vi "BS the tug main A.vi"() -> ()   [LabVIEW 2012]
uses:
  <vilib>/userdefined/High Color/IMAQdx.ctl
  <vilib>/vision/driver/NI_Vision_Acquisition_Software.lvlib
  <vilib>/vision/NI_Vision_Development_Module.lvlib
panel:
  out "Scaled image":T1(plugin-control)
  out "Running?":bool
  out "All found?":bool
  in  "Data sent":string
  out "error out":errorcluster
  out "Image":T1(plugin-control)
  in  "stop":bool
  in  "Image Type":T2 items=["Grayscale (U8)", "Grayscale (I16)", "Grayscale (SGL)", "Complex (CSG)", "RGB (U32)", "HSL (U32)", "RGB (U64)", "Grayscale (U16)"]
  in  "Session In":T3="cam0"
  # "This VI receives an image from the camera above the pool and modifies the image to be 1032 x 1032 it then:\n1. Locates (4) tugs with greek letter symbols\n2. Locates (4) buoys with circle symbols\n3. Records the time the image is taken\n4. Creates a single string of that data and transmits the string using UDP to port 61557\n\nTO OPERATE START THE ROUTINE!"
  # "The Point Grey camera settings should be:\nAuto Exposure      Auto\nBrightness             Relative     200\nGain                       Auto\nFrame Rate           Absolute   20\nShutter                  Auto\n\nThese values are programmed into this VI\n\nThe overhead lights should be OFF"
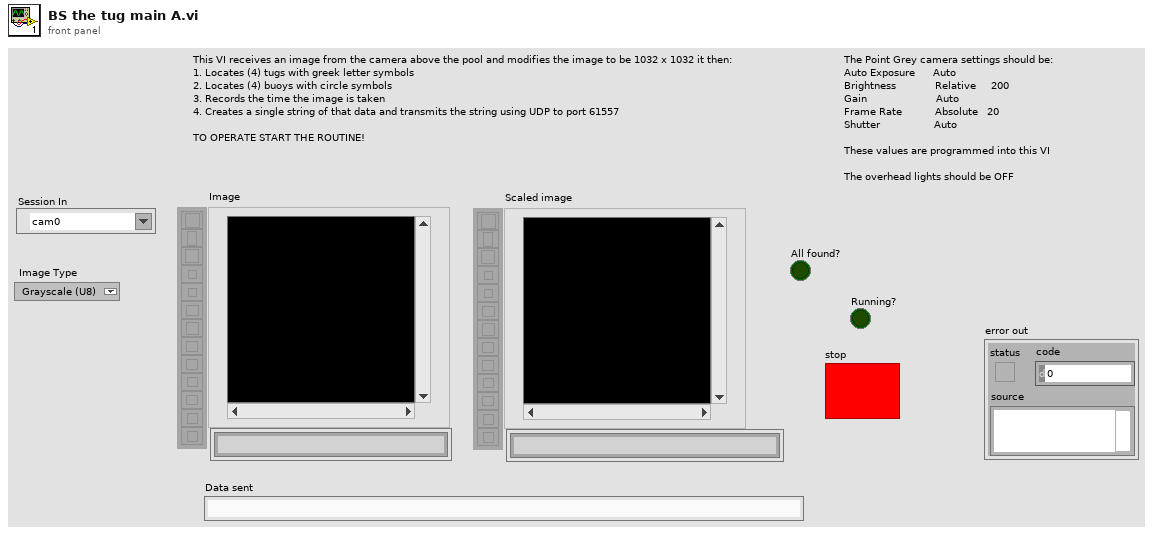
[diagram p1: front panel]
types:
  T1 = typedef "IMAQ Image.ctl" = refnum<image>
  T2 = typedef "Image Type" = u32
  T3 = typedef "IMAQdx.ctl" = refnum<k21>
  T4 = cluster{"Greek Letter":string, i16, i16, i16, bool}[]
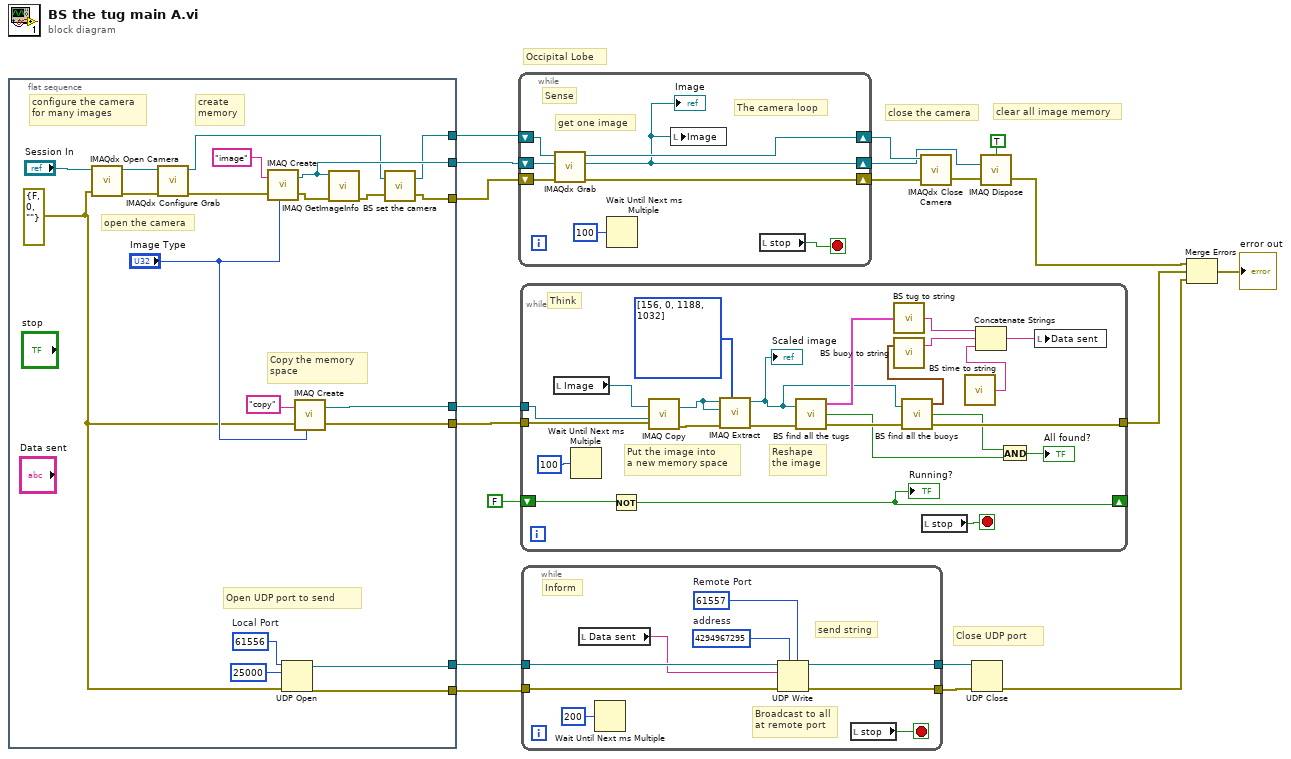
[diagram p0: block diagram]
diagram:
  # "Occipital Lobe"
  # "Close UDP port"
  # "clear all image memory"
  # "close the camera"
  n1 = flat-sequence {
    tunnel: [w22] -> w12
    tunnel: [w20] -> w13
    tunnel: [w33] -> w14
    tunnel: [w30] -> w10
    tunnel: [w29] -> w11
    tunnel: [w26] -> w4
    tunnel: [w25] -> w3
    frame #0 {
      w28 = u16 61556  # Local Port
      w24 = errorcluster {"status"=FALSE, "code"=0, "source"=""} ("error in")
      # "Open UDP port to send"
      # "Copy the memory\nspace"
      # "create\nmemory"
      # "configure the camera\nfor many images"
      # "open the camera"
      n2 = call <vilib>:"IMAQdx Open Camera.vi"("error in"=w24, "Session In"="Session In") -> ("error out"=w36:errorcluster, "Session Out"=w37:T3)  [unwired: 1 in, 7 out]
      n3 = call <vilib>:"IMAQdx Configure Grab.vi"("error in"=w36, "Session In"=w37) -> ("error out"=w38:errorcluster, "Session Out"=w21:T3)  [unwired: 8 out]
      n4 = call "IMAQ Create"("Image Name"="image", "Image Type"="Image Type", "error in (no error)"=w38) -> ("New Image"=w33:T1, "error out"=w39:errorcluster)  [unwired: 1 in, 1 out]
      n5 = UDP Open(8:w24, 9:25000 ("timeout ms (25000)"), 11:w28) -> (port=w25:refnum<k16>, 0:w26:errorcluster)  [unwired: 3 out]
      n6 = call "IMAQ Create"("Image Name"="copy", "Image Type"="Image Type", "error in (no error)"=w24) -> ("New Image"=w29:T1, "error out"=w30:errorcluster)  [unwired: 2 in]
      n7 = call "IMAQ GetImageInfo"("error in (no error)"=w39, "Image"=w33) -> ("error out"=w23:errorcluster)  [unwired: 2 in, 7 out]
      n8 = call "BS set the camera.vi"("error in"=w23, "IMAQdx Session input"=w21) -> ("error out"=w22:errorcluster, "IMAQdx Session output"=w20:T3)
    }
  }
  n9 = while {
    shift-right: [w44] -> w19
    shift-left: w13 -> [w47]
    shift-right: [w40] -> w16
    shift-left: w14 -> [w46]
    shift-right: [w43] -> w18
    shift-left: w12 -> [w45]
    stop <- w41 stop-if-true
    # "Sense"
    # "The camera loop"
    # "get one image"
    n10 = call <vilib>:"IMAQdx Grab.vi"("error in"=w45, "Image In"=w46, "Session In"=w47) -> ("error out"=w43:errorcluster, "Image Out"=w40:T1, "Session Out"=w44:T3)  [unwired: 5 in, 1 out]
    "Image" <- w40
    n11 = Wait Until Next ms Multiple(millisecond multiple=u32 100) -> ()  [unwired: 1 out]
    n12 = local write "Image"(w40) -> ()
    n13 = local read "stop"() -> (w41:bool)
  }
  n14 = while {
    tunnel: w11 -> [w66]
    tunnel: w10 -> [w67]
    tunnel: [w56] -> w8
    shift-right: [w59] -> _
    shift-left: FALSE -> [w60]
    stop <- w62 stop-if-true
    # "Think"
    # "Reshape\nthe image"
    # "Put the image into \na new memory space"
    n15 = local read "Image"() -> (w65:T1)
    n16 = Wait Until Next ms Multiple(millisecond multiple=u32 100) -> ()  [unwired: 1 out]
    n17 = Not(x=w60) -> (.not. x?=w59:bool)
    "Running?" <- w59
    n18 = call "IMAQ Copy"("error in (no error)"=w67, "Image Dst"=w66, "Image Src"=w65) -> ("error out"=w69:errorcluster, "Image Dst Out"=w70:T1)  [unwired: 3 in]
    n19 = call "IMAQ Extract"("Optional Rectangle"=i32[] [156, 0, 1188, 1032], "error in (no error)"=w69, "Image Dst"=w70, "Image Src"=w70) -> ("error out"=w64:errorcluster, "Image Dst Out"=w57:T1)  [unwired: 6 in]
    "Scaled image" <- w57
    n20 = call "BS find all the tugs.vi"("Image Src"=w57, "error in"=w64) -> ("Tug location array"=w63:T4, "All found?"=w52:bool, "error out"=w58:errorcluster)
    n21 = call "BS tug to string.vi"("Tug location array"=w63) -> ("tug location string"=w51:string)
    n22 = call "BS find all the buoys.vi"("Image Src"=w57, "error in"=w58) -> ("Buoy Array"=w54:cluster{i16, i16}[], "Buoys found?"=w53:bool, "error out"=w56:errorcluster)
    n23 = call "BS buoy to string.vi"("Buoy Array"=w54) -> ("Buoy location string"=w50:string)  [unwired: 1 in, 1 out]
    n24 = local read "stop"() -> (w62:bool)
    n25 = call "BS time to string.vi"() -> ("time string"=w49:string)  [unwired: 1 in]
    n26 = Concatenate Strings(w51, w50, w49) -> (w48:string)
    n27 = And(x=w53, y=w52) -> (x .and. y?=→"All found?":bool)
    n28 = local write "Data sent"(w48) -> ()
  }
  n29 = while {
    tunnel: w3 -> [w79]
    tunnel: w4 -> [w78]
    tunnel: [w77] -> w6
    tunnel: [w76] -> w5
    stop <- w72 stop-if-true
    w75 = u16 61557  # Remote Port
    w74 = u32 4294967295  # address
    # "Inform"
    # "send string"
    # "Broadcast to all\nat remote port"
    n30 = local read "Data sent"() -> (w73:string)
    n31 = Wait Until Next ms Multiple(millisecond multiple=u32 200) -> ()  [unwired: 1 out]
    n32 = UDP Write(address=w74, port or service name=w75, connection ID=w79, data in=w73, 8:w78) -> (error out=w77:errorcluster, 3:w76:refnum<k16>)  [unwired: 1 out]
    n33 = local read "stop"() -> (w72:bool)
  }
  n34 = call <vilib>:"IMAQdx Close Camera.vi"("error in"=w18, "Session In"=w19) -> ("error out"=w17:errorcluster)  [unwired: 9 out]
  n35 = UDP Close(connection ID=w5, 8:w6) -> (error out=w2:errorcluster)  [unwired: 1 out]
  n36 = call "IMAQ Dispose"("All Images? (No)"=TRUE, "Image"=w16, "error in (no error)"=w17) -> ("error out"=w9:errorcluster)  [unwired: 3 out]
  n37 = Merge Errors(w9, w8, w2) -> (→"error out":errorcluster)
